vi "Begin.vi"() -> (0 "error out":errorcluster)   [LabVIEW 2013]
doc: "Called before other user functions, this VI is expected to open initial I/O refnums, load in file data, and do all program initialization. Notice that the <B>error out</B> terminal is simply used for data flow. Wiring it to other structures or subVIs ensures that this VI runs first."
uses:
  <vilib>/Rock Robotics/WPI/SafetyOutput/WPI_SafetyOutputConfigMenu.ctl
  <vilib>/Rock Robotics/WPI/DriverStation/WPI_DriverStationRobotMode2.ctl
  <vilib>/Rock Robotics/WPI/Joystick/WPI_JoystickDeviceEnum.ctl
  <vilib>/Rock Robotics/SystemInterfaces/DIO/FPGA_DIOChannel.ctl
  <vilib>/Rock Robotics/WPI/Solenoid/WPI_SolenoidChannel.ctl
  <vilib>/Rock Robotics/SystemInterfaces/DIO/FPGA_DIORelayChannel.ctl
  <vilib>/Rock Robotics/SystemInterfaces/AI/FPGA_AIChannel.ctl
  Robot Global Data.vi
  <vilib>/Rock Robotics/WPI/Counter/WPI_CounterDigitalInputToDigitalSource.vi
  <vilib>/Rock Robotics/WPI/Solenoid/WPI_SolenoidOpenSingle.vi
  <vilib>/Rock Robotics/WPI/RobotDrive/WPI_RobotDriveOpen4MotorWithCANJaguar.vi
  <vilib>/Rock Robotics/WPI/Solenoid/WPI_SolenoidOpenDouble.vi
  <vilib>/Rock Robotics/WPI/MotorControl/WPI_MotorControlOpenCANJaguar.vi
  <vilib>/Rock Robotics/WPI/Compressor/WPI_CompressorGetSetRefNum.vi
panel:
  out "error out 2":errorcluster
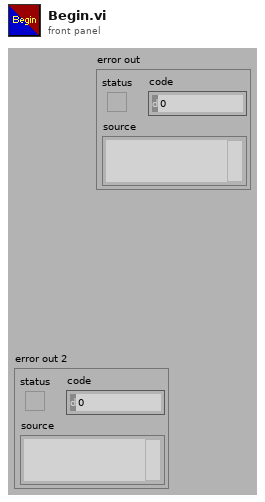
[diagram p1: front panel]
types:
  T1 = typedef "FPGA_DIOChannel.ctl" = enum8{"DIO 1", "DIO 2", "DIO 3", "DIO 4", "DIO 5", "DIO 6", "DIO 7", "DIO 8", "DIO 9", "DIO 10", "DIO 11", "DIO 12", "DIO 13", "DIO 14", "Invalid"}
  T2 = typedef "FPGA_DIORelayChannel.ctl" = enum8{"Relay 1", "Relay 2", "Relay 3", "Relay 4", "Relay 5", "Relay 6", "Relay 7", "Relay 8", "Invalid"}
  T3 = typedef "FPGA_AIChannel.ctl" = enum8{"AI 1", "AI 2", "AI 3", "AI 4", "AI 5", "AI 6", "AI 7", "AI 8", "Invalid"}
  T4 = typedef "WPI_SolenoidChannel.ctl" = enum8{"Solenoid 1", "Solenoid 2", "Solenoid 3", "Solenoid 4", "Solenoid 5", "Solenoid 6", "Solenoid 7", "Solenoid 8", "Invalid"}
  T5 = typedef "WPI_JoystickDeviceEnum.ctl" = enum16{"USB 1", "USB 2", "USB 3", "USB 4", "Kinect 1", "Kinect 2"}
  T6 = typedef "WPI_DriverStationRobotMode2.ctl" = enum16{"Autonomous Disabled", "Autonomous Enabled", "Teleop Disabled", "Teleop Enabled", "Timeout", "Finish", "Test Disabled", "Test Enabled"}
  T7 = typedef "WPI_SafetyOutputConfigMenu.ctl" = enum16{"Enable", "Disable"}
  T8 = typedef "WPI_DigitalInputDevRef.ctl" = cluster{"DevStatus":errorcluster, "DIO Channel":T1, "Digital Module":T9}
  T9 = typedef "FPGA_TypedefDigitalModule.ctl" = enum16{"Digital Module 1", "Digital Module 2"}
  T10 = typedef "FPGA_CounterEncoderSourceConvertionLVSourceType.ctl" = cluster{"DevStatus":errorcluster, "AnalogTriggerMode?":bool, "DigitalMode":cluster{"Digital Module":T9, "DIO Channel":T11}, "AnalogTriggerMode":cluster{"AnalogTriggerIndex":T12, "OutputType":T13}}
  T11 = typedef "FPGA_DIODigitalSourceChannel.ctl" = enum8{"DIO 1", "DIO 2", "DIO 3", "DIO 4", "DIO 5", "DIO 6", "DIO 7", "DIO 8", "DIO 9", "DIO 10", "DIO 11", "DIO 12", "DIO 13", "DIO 14", "Disabled"}
  T12 = typedef "FPGA_AnalogTriggerIndex.ctl" = enum8{"Trig 0", "Trig 1", "Trig 2", "Trig 3", "Trig 4", "Trig 5", "Trig 6", "Trig 7", "Invalid"}
  T13 = typedef "FPGA_AnalogTriggerOutType.ctl" = enum16{"InWindow", "TriggerState", "Rising", "Falling"}
  T14 = typedef "WPI_JoystickDevRef.ctl" = cluster{"Device":T5}
  T15 = typedef "WPI_RobotDriveDevRef.ctl" = cluster{"DevStatus":errorcluster, "Motors[]":T16[], "Square Inputs":bool, "Max Output":dbl, "Isochronous":bool}
  T16 = typedef "WPI_MotorControlDeviceRef.ctl" = cluster{"DeviceStatus":errorcluster, "Type":enum16{"PWM", "CAN"}, "PWM":cluster{"Digital Module":T9, "PWM Channel":T17, "DeadBand":T18}, "CAN":cluster{"Device Number":u8, "Control Mode":T19, "Semaphore":T20, "Max Vout":dbl}, "Invert":bool, "TransformRef":T21, "InvTransformRef":T21}
  T17 = typedef "FPGA_DIOPWMChannel.ctl" = enum8{"PWM 1", "PWM 2", "PWM 3", "PWM 4", "PWM 5", "PWM 6", "PWM 7", "PWM 8", "PWM 9", "PWM 10", "Invalid"}
  T18 = typedef "WPI_PWMDeadband.ctl" = cluster{"Name":string, "maxPositivePwm":i32, "minPositivePwm":i32, "centerPwm":i32, "maxNegativePwm":i32, "minNegativePwm":i32, "angularRange":u16}
  T19 = typedef "WPI_CANJaguar_ControlMode.ctl" = enum8{"Percent VBus", "Current", "Speed", "Position", "Voltage"}
  T20 = typedef "Semaphore RefNum" = refnum<k1>
  T21 = typedef "WPI_PWMTransform_ConPane.ctl" = refnum<vi>
  T22 = typedef "WPI_EncoderDevRef.ctl" = cluster{"DevStatus":errorcluster, "EncoderIndex":T23, "CounterIndex":T24, "DistancePerCount":dbl, "Decoding Type":T25}
  T23 = typedef "FPGA_EncoderIdx.ctl" = enum8{"Enc 0", "Enc 1", "Enc 2", "Enc 3", "Invalid"}
  T24 = typedef "FPGA_CounterCtrSystemIndex.ctl" = enum8{"Ctr 0", "Ctr 1", "Ctr 2", "Ctr 3", "Ctr 4", "Ctr 5", "Ctr 6", "Ctr 7", "Invalid"}
  T25 = typedef "WPI_EncoderType.ctl" = enum16{"1x", "2x", "4x"}
  T26 = typedef "WPI_AnalogChannelDevRef.ctl" = cluster{"DevStatus":errorcluster, "Analog Module":T27, "Analog Channel":T3}
  T27 = typedef "FPGA_TypedefAnalogModule.ctl" = enum16{"Analog Module 1", "Analog Module 2"}
  T28 = typedef "WPI_CompressorDevRef.ctl" = cluster{"DevStatus":errorcluster, "DigitalInputDevRef":T8, "RelayDevRef":T29}
  T29 = typedef "WPI_RelayDevRef.ctl" = cluster{"DevStatus":errorcluster, "Relay Channel":T2, "Digital Module":T9, "Relay Direction":T30}
  T30 = typedef "WPI_RelayDirection.ctl" = enum16{"Both directions", "Forward only", "Reverse only"}
  T31 = typedef "WPI_SolenoidDevRef.ctl" = cluster{"DevStatus":errorcluster, "Solenoid Module":T32, "Forward Solenoid Channel":T4, "Reverse Solenoid Channel":T4}
  T32 = typedef "FPGA_TypedefSolenoidModule.ctl" = enum16{"Solenoid Module 1", "Solenoid Module 2"}
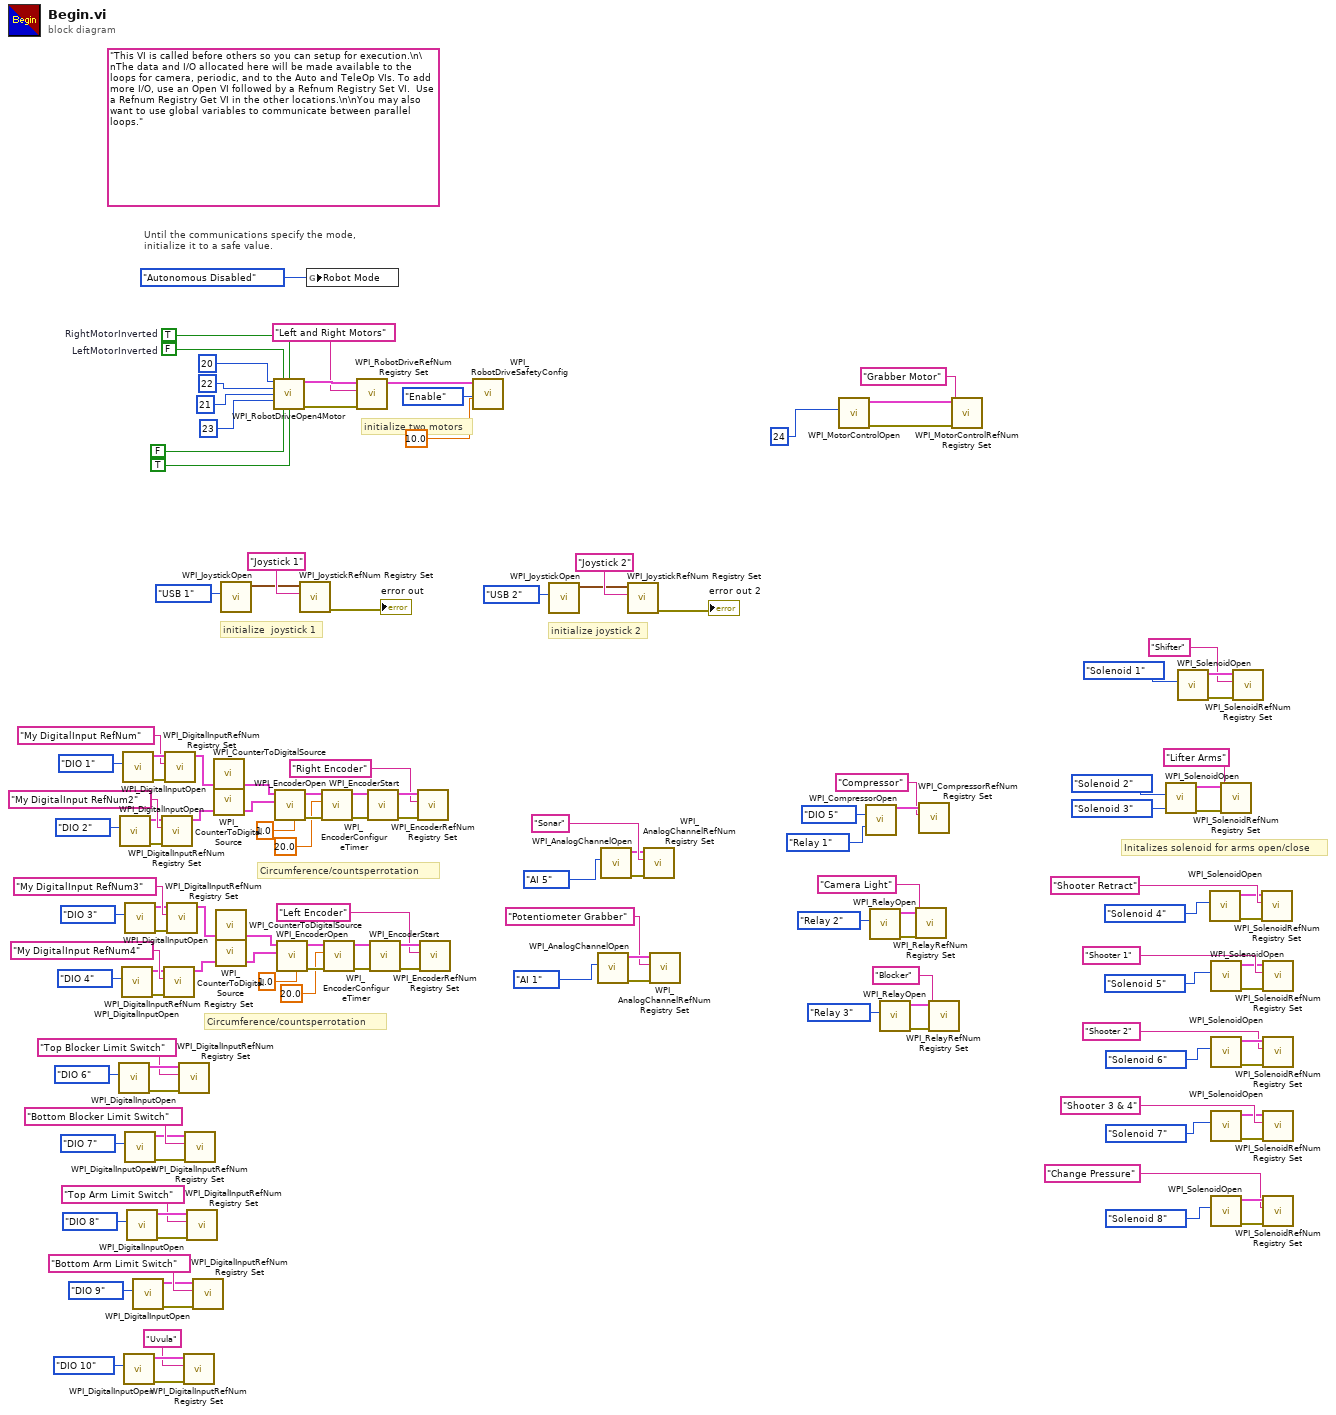
[diagram p0: block diagram]
diagram:
  (unwired) "This VI is called before others so you can setup for execution.\n\nThe data and I/O allocated here will be made available to the loops for camera, periodic, and to the Auto and TeleOp VIs. To add more I/O, use an Open VI followed by a Refnum Registry Set VI.  Use a Refnum Registry Get VI in the other locations.\n\nYou may also want to use global variables to communicate between parallel loops."
  w81 = FALSE  # LeftMotorInverted
  w80 = TRUE  # RightMotorInverted
  # "Initalizes solenoid for arms open/close"
  # "initialize joystick 2"
  # "Circumference/countsperrotation"
  # "Circumference/countsperrotation"
  # "initialize  joystick 1"
  # "Until the communications specify the mode,\ninitialize it to a safe value."
  # "initialize two motors"
  n1 = call <vilib>:"WPI_DigitalInputOpen.vi"("DIO Channel"=FPGA_DIOChannel."DIO 6") -> ("error out"=w18:errorcluster, "DigitalInputDevRef"=w17:T8)  [unwired: 9 in]
  n2 = call <vilib>:"WPI_DigitalInputOpen.vi"("DIO Channel"=FPGA_DIOChannel."DIO 2") -> ("error out"=w110:errorcluster, "DigitalInputDevRef"=w111:T8)  [unwired: 9 in]
  n3 = call <vilib>:"WPI_DigitalInputOpen.vi"("DIO Channel"=FPGA_DIOChannel."DIO 4") -> ("error out"=w105:errorcluster, "DigitalInputDevRef"=w43:T8)  [unwired: 9 in]
  n4 = call <vilib>:"WPI_DigitalInputOpen.vi"("DIO Channel"=FPGA_DIOChannel."DIO 1") -> ("error out"=w119:errorcluster, "DigitalInputDevRef"=w118:T8)  [unwired: 9 in]
  n5 = call <vilib>:"WPI_DigitalInputOpen.vi"("DIO Channel"=FPGA_DIOChannel."DIO 10") -> ("error out"=w10:errorcluster, "DigitalInputDevRef"=w9:T8)  [unwired: 9 in]
  n6 = call <vilib>:"WPI_DigitalInputOpen.vi"("DIO Channel"=FPGA_DIOChannel."DIO 3") -> ("error out"=w97:errorcluster, "DigitalInputDevRef"=w98:T8)  [unwired: 9 in]
  n7 = call <vilib>:"WPI_DigitalInputOpen.vi"("DIO Channel"=FPGA_DIOChannel."DIO 7") -> ("error out"=w11:errorcluster, "DigitalInputDevRef"=w12:T8)  [unwired: 9 in]
  n8 = call <vilib>:"WPI_DigitalInputOpen.vi"("DIO Channel"=FPGA_DIOChannel."DIO 8") -> ("error out"=w30:errorcluster, "DigitalInputDevRef"=w29:T8)  [unwired: 9 in]
  n9 = call <vilib>:"WPI_DigitalInputOpen.vi"("DIO Channel"=FPGA_DIOChannel."DIO 9") -> ("error out"=w23:errorcluster, "DigitalInputDevRef"=w24:T8)  [unwired: 9 in]
  n10 = call <vilib>:"WPI_DigitalInputRefNum Registry Set.vi"("error in (no error)"=w110, "refnum name"="My DigitalInput RefNum2", "DigitalInputDevRef"=w111) -> ("DigitalInputDevRef"=w109:T8)  [unwired: 7 in, 1 out]
  n11 = call <vilib>:"WPI_DigitalInputRefNum Registry Set.vi"("error in (no error)"=w105, "refnum name"="My DigitalInput RefNum4", "DigitalInputDevRef"=w43) -> ("DigitalInputDevRef"=w106:T8)  [unwired: 7 in, 1 out]
  n12 = call <vilib>:"WPI_DigitalInputRefNum Registry Set.vi"("error in (no error)"=w119, "refnum name"="My DigitalInput RefNum", "DigitalInputDevRef"=w118) -> ("DigitalInputDevRef"=w117:T8)  [unwired: 7 in, 1 out]
  n13 = call <vilib>:"WPI_DigitalInputRefNum Registry Set.vi"("error in (no error)"=w97, "refnum name"="My DigitalInput RefNum3", "DigitalInputDevRef"=w98) -> ("DigitalInputDevRef"=w99:T8)  [unwired: 7 in, 1 out]
  n14 = call <vilib>:"WPI_DigitalInputRefNum Registry Set.vi"("error in (no error)"=w18, "refnum name"="Top Blocker Limit Switch", "DigitalInputDevRef"=w17) -> ()  [unwired: 7 in, 2 out]
  n15 = call <vilib>:"WPI_DigitalInputRefNum Registry Set.vi"("error in (no error)"=w10, "refnum name"="Uvula", "DigitalInputDevRef"=w9) -> ()  [unwired: 7 in, 2 out]
  n16 = call <vilib>:"WPI_DigitalInputRefNum Registry Set.vi"("error in (no error)"=w11, "refnum name"="Bottom Blocker Limit Switch", "DigitalInputDevRef"=w12) -> ()  [unwired: 7 in, 2 out]
  n17 = call <vilib>:"WPI_DigitalInputRefNum Registry Set.vi"("error in (no error)"=w30, "refnum name"="Top Arm Limit Switch", "DigitalInputDevRef"=w29) -> ()  [unwired: 7 in, 2 out]
  n18 = call <vilib>:"WPI_DigitalInputRefNum Registry Set.vi"("error in (no error)"=w23, "refnum name"="Bottom Arm Limit Switch", "DigitalInputDevRef"=w24) -> ()  [unwired: 7 in, 2 out]
  n19 = call-poly <vilib>:"WPI_CounterToDigitalSource.vi"("DigitalInputDevRef"=w117) -> ("Digital Source"=w120:T10)  [unwired: 6 in]
  n20 = call-poly <vilib>:"WPI_CounterToDigitalSource.vi"("DigitalInputDevRef"=w109) -> ("Digital Source"=w115:T10)  [unwired: 6 in]
  n21 = call-poly <vilib>:"WPI_CounterToDigitalSource.vi"("DigitalInputDevRef"=w99) -> ("Digital Source"=w96:T10)  [unwired: 6 in]
  n22 = call-poly <vilib>:"WPI_CounterToDigitalSource.vi"("DigitalInputDevRef"=w106) -> ("Digital Source"=w101:T10)  [unwired: 6 in]
  n23 = call <vilib>:"WPI_JoystickOpen.vi"("JoystickDevice"=WPI_JoystickDeviceEnum."USB 1") -> ("JoystickDevRef"=w132:T14)  [unwired: 10 in]
  n24 = call-poly <vilib>:"WPI_RobotDriveOpen4Motor.vi"("Rear Left Motor"=u8 20, "Rear Left Motor Inverted"=w81, "Rear Right Motor Inverted"=w80, "Rear Right Motor"=u8 22, "Front Left Motor"=u8 21, "Front Right Motor"=u8 23, "Front Left Motor Inverted"=FALSE, "Front Right Motor Inverted"=TRUE) -> ("RobotDriveDevRef"=w138:T15, "error out"=w136:errorcluster)  [unwired: 6 in]
  n25 = call <vilib>:"WPI_EncoderOpen.vi"("DistancePerCount"=1.0, "BSource"=w115, "ASource"=w120) -> ("error out"=w126:errorcluster, "EncoderDevRef"=w125:T22)  [unwired: 7 in]
  n26 = call <vilib>:"WPI_EncoderOpen.vi"("DistancePerCount"=1.0, "BSource"=w101, "ASource"=w96) -> ("error out"=w90:errorcluster, "EncoderDevRef"=w91:T22)  [unwired: 7 in]
  n27 = call <vilib>:"WPI_JoystickRefNum Registry Set.vi"("refnum name"="Joystick 1", "JoystickDevRef"=w132) -> ("error out"=→"error out":errorcluster)  [unwired: 8 in, 1 out]
  n28 = global write "Robot Global Data.vi" "Robot Mode"(WPI_DriverStationRobotMode2."Autonomous Disabled" ("Robot Mode")) -> ()
  n29 = call <vilib>:"WPI_EncoderConfigureTimer.vi"("error in (no error)"=w126, "Minimum Rate"=20.0, "EncoderDevRef"=w125) -> ("error out"=w124:errorcluster, "EncoderDevRef"=w123:T22)  [unwired: 7 in]
  n30 = call <vilib>:"WPI_EncoderConfigureTimer.vi"("error in (no error)"=w90, "Minimum Rate"=20.0, "EncoderDevRef"=w91) -> ("error out"=w92:errorcluster, "EncoderDevRef"=w93:T22)  [unwired: 7 in]
  n31 = call <vilib>:"WPI_RobotDriveRefNum Registry Set.vi"("error in (no error)"=w136, "refnum name"="Left and Right Motors", "RobotDriveDevRef"=w138) -> ("RobotDriveDevRef"=w4:T15)  [unwired: 8 out]
  n32 = call <vilib>:"WPI_EncoderStart.vi"("error in (no error)"=w124, "EncoderDevRef"=w123) -> ("error out"=w122:errorcluster, "EncoderDevRef"=w121:T22)  [unwired: 8 in]
  n33 = call <vilib>:"WPI_EncoderStart.vi"("error in (no error)"=w92, "EncoderDevRef"=w93) -> ("error out"=w94:errorcluster, "EncoderDevRef"=w95:T22)  [unwired: 8 in]
  n34 = call <vilib>:"WPI_EncoderRefNum Registry Set.vi"("error in (no error)"=w122, "refnum name"="Right Encoder", "EncoderDevRef"=w121) -> ()  [unwired: 7 in, 2 out]
  n35 = call <vilib>:"WPI_EncoderRefNum Registry Set.vi"("error in (no error)"=w94, "refnum name"="Left Encoder", "EncoderDevRef"=w95) -> ()  [unwired: 7 in, 2 out]
  n36 = call <vilib>:"WPI_RobotDriveSafetyConfig.vi"("timeout (s)"=10.0, "mode"=WPI_SafetyOutputConfigMenu."Enable", "RobotDriveDevRef"=w4) -> ()  [unwired: 7 in, 2 out]
  n37 = call <vilib>:"WPI_JoystickOpen.vi"("JoystickDevice"=WPI_JoystickDeviceEnum."USB 2") -> ("JoystickDevRef"=w66:T14)  [unwired: 10 in]
  n38 = call <vilib>:"WPI_AnalogChannelOpen.vi"("Analog Channel"=FPGA_AIChannel."AI 1") -> ("error out"=w63:errorcluster, "AIDeviceRef"=w62:T26)  [unwired: 9 in]
  n39 = call <vilib>:"WPI_AnalogChannelOpen.vi"("Analog Channel"=FPGA_AIChannel."AI 5") -> ("error out"=w31:errorcluster, "AIDeviceRef"=w32:T26)  [unwired: 9 in]
  n40 = call <vilib>:"WPI_JoystickRefNum Registry Set.vi"("refnum name"="Joystick 2", "JoystickDevRef"=w66) -> ("error out"=→"error out 2":errorcluster)  [unwired: 8 in, 1 out]
  n41 = call <vilib>:"WPI_AnalogChannelRefNum Registry Set.vi"("error in (no error)"=w31, "refnum name"="Sonar", "AIDeviceRef"=w32) -> ()  [unwired: 7 in, 2 out]
  n42 = call <vilib>:"WPI_AnalogChannelRefNum Registry Set.vi"("error in (no error)"=w63, "refnum name"="Potentiometer Grabber", "AIDeviceRef"=w62) -> ()  [unwired: 7 in, 2 out]
  n43 = call-poly <vilib>:"WPI_MotorControlOpen.vi"("Device Number"=u8 24) -> ("error out"=w2:errorcluster, "MotorControlDeviceRef"=w3:T16)  [unwired: 9 in]
  n44 = call <vilib>:"WPI_CompressorOpen.vi"("Pressure Switch DIO Channel"=FPGA_DIOChannel."DIO 5", "Relay Channel"=FPGA_DIORelayChannel."Relay 1") -> ("CompressorDevRef"=w69:T28)  [unwired: 12 in, 1 out]
  n45 = call <vilib>:"WPI_RelayOpen.vi"("Relay Channel"=FPGA_DIORelayChannel."Relay 2") -> ("error out"=w42:errorcluster, "RelayDevRef"=w41:T29)  [unwired: 9 in]
  n46 = call <vilib>:"WPI_RelayOpen.vi"("Relay Channel"=FPGA_DIORelayChannel."Relay 3") -> ("error out"=w22:errorcluster, "RelayDevRef"=w21:T29)  [unwired: 9 in]
  n47 = call <vilib>:"WPI_RelayRefNum Registry Set.vi"("error in (no error)"=w42, "refnum name"="Camera Light", "RelayDevRef"=w41) -> ()  [unwired: 7 in, 2 out]
  n48 = call <vilib>:"WPI_CompressorRefNum Registry Set.vi"("refnum name"="Compressor", "CompressorDevRef"=w69) -> ()  [unwired: 8 in, 2 out]
  n49 = call <vilib>:"WPI_RelayRefNum Registry Set.vi"("error in (no error)"=w22, "refnum name"="Blocker", "RelayDevRef"=w21) -> ()  [unwired: 7 in, 2 out]
  n50 = call <vilib>:"WPI_MotorControlRefNum Registry Set.vi"("error in (no error)"=w2, "refnum name"="Grabber Motor", "MotorControlDevRef"=w3) -> ()  [unwired: 7 in, 2 out]
  n51 = call-poly <vilib>:"WPI_SolenoidOpen.vi"("Reverse Solenoid Channel"=WPI_SolenoidChannel."Solenoid 3", "Forward Solenoid Channel"=WPI_SolenoidChannel."Solenoid 2") -> ("error out"=w73:errorcluster, "SolenoidDevRef"=w74:T31)  [unwired: 8 in]
  n52 = call-poly <vilib>:"WPI_SolenoidOpen.vi"("Solenoid Channel"=WPI_SolenoidChannel."Solenoid 1" ("Forward Solenoid Channel")) -> ("error out"=w85:errorcluster, "SolenoidDevRef"=w84:T31)  [unwired: 9 in]
  n53 = call-poly <vilib>:"WPI_SolenoidOpen.vi"("Solenoid Channel"=WPI_SolenoidChannel."Solenoid 4" ("Forward Solenoid Channel")) -> ("error out"=w35:errorcluster, "SolenoidDevRef"=w36:T31)  [unwired: 9 in]
  n54 = call-poly <vilib>:"WPI_SolenoidOpen.vi"("Solenoid Channel"=WPI_SolenoidChannel."Solenoid 5" ("Forward Solenoid Channel")) -> ("error out"=w56:errorcluster, "SolenoidDevRef"=w57:T31)  [unwired: 9 in]
  n55 = call-poly <vilib>:"WPI_SolenoidOpen.vi"("Solenoid Channel"=WPI_SolenoidChannel."Solenoid 6" ("Forward Solenoid Channel")) -> ("error out"=w51:errorcluster, "SolenoidDevRef"=w50:T31)  [unwired: 9 in]
  n56 = call-poly <vilib>:"WPI_SolenoidOpen.vi"("Solenoid Channel"=WPI_SolenoidChannel."Solenoid 7" ("Forward Solenoid Channel")) -> ("error out"=w44:errorcluster, "SolenoidDevRef"=w45:T31)  [unwired: 9 in]
  n57 = call-poly <vilib>:"WPI_SolenoidOpen.vi"("Solenoid Channel"=WPI_SolenoidChannel."Solenoid 8" ("Forward Solenoid Channel")) -> ("error out"=w55:errorcluster, "SolenoidDevRef"=w54:T31)  [unwired: 9 in]
  n58 = call <vilib>:"WPI_SolenoidRefNum Registry Set.vi"("error in (no error)"=w73, "refnum name"="Lifter Arms", "SolenoidDevRef"=w74) -> ()  [unwired: 7 in, 2 out]
  n59 = call <vilib>:"WPI_SolenoidRefNum Registry Set.vi"("error in (no error)"=w85, "refnum name"="Shifter", "SolenoidDevRef"=w84) -> ()  [unwired: 7 in, 2 out]
  n60 = call <vilib>:"WPI_SolenoidRefNum Registry Set.vi"("error in (no error)"=w35, "refnum name"="Shooter Retract", "SolenoidDevRef"=w36) -> ()  [unwired: 7 in, 2 out]
  n61 = call <vilib>:"WPI_SolenoidRefNum Registry Set.vi"("error in (no error)"=w56, "refnum name"="Shooter 1", "SolenoidDevRef"=w57) -> ()  [unwired: 7 in, 2 out]
  n62 = call <vilib>:"WPI_SolenoidRefNum Registry Set.vi"("error in (no error)"=w51, "refnum name"="Shooter 2", "SolenoidDevRef"=w50) -> ()  [unwired: 7 in, 2 out]
  n63 = call <vilib>:"WPI_SolenoidRefNum Registry Set.vi"("error in (no error)"=w44, "refnum name"="Shooter 3 & 4", "SolenoidDevRef"=w45) -> ()  [unwired: 7 in, 2 out]
  n64 = call <vilib>:"WPI_SolenoidRefNum Registry Set.vi"("error in (no error)"=w55, "refnum name"="Change Pressure", "SolenoidDevRef"=w54) -> ()  [unwired: 7 in, 2 out]
